vi "ATS_GetASOPC.vi"(11 "DeviceIn":i32) -> (0 "Minor":u32, 1 "Major":u32, 2 "ASoPC":string, 4 "ReturnValue":u32)   [LabVIEW 2014]
doc: "_____AlazarTech, Scope_____\n\nRetrieve the CPLG version number.\n\nInput:\n\"HandleIn\" = device to retrieve information\n\nOutput:\n\"HandleOut\" = device information\n\"Version\" = version\n\"Board\" = board name\n\"ID\" = board identification"
uses:
  ATS_ctl/ATS_Global_Ctrl.ctl
  ATS_ctl/ATS_Query.ctl
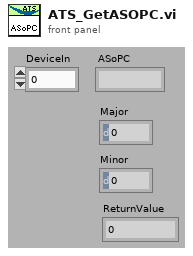
[diagram p1: front panel]
types:
  T1 = typedef "ATS_Query.ctl" = enum16{"None", "NUMBER_OF_RECORDS", "PRETRIGGER_AMOUNT", "RECORD_LENGTH", "TRIGGER_ENGINE", "TRIGGER_DELAY", "TRIGGER_TIMEOUT", "SAMPLE_RATE", "CONFIGURATION_MODE", "DATA_WIDTH", "AUTO_CALIBRATE", "TRIGGER_XXXXX", "CLOCK_SOURCE", "CLOCK_SLOPE", "IMPEDANCE", "INPUT_RANGE", "COUPLING", "MAX_TIMEOUTS_ALLOWED", "ATS_OPERATING_MODE", "CLOCK_DECIMATION_EXTERNAL", "LED_CONTROL", "ATTENUATOR_RELAY", "EXT_TRIGGER_COUPLING", "EXT_TRIGGER_ATTENUATOR_RELAY", "TRIGGER_ENGINE_SOURCE", "TRIGGER_ENGINE_SLOPE", "SEND_DAC_VALUE", "SLEEP_DEVICE", "MEMORY_SIZE", "BOARD_TYPE", "ASOPC_TYPE", "SERIAL_NUMBER", "FIRSTCAL_DATE", "LATEST_CAL_DATE", "LATEST_TEST_DATE"}
  T2 = typedef "ATS_Global_Ctrl.ctl" = enum16{"Init_Device", "Clear_ALL", "Set", "Get"}
  T3 = typedef "Device_Info.ctl" = cluster{"Handle":u32, "Board":string, "CPLD":string, "MemorySize":u32, "SampleSize":u8, "ID":i32, "High_Memory":bool, "Chan/Board":u8}
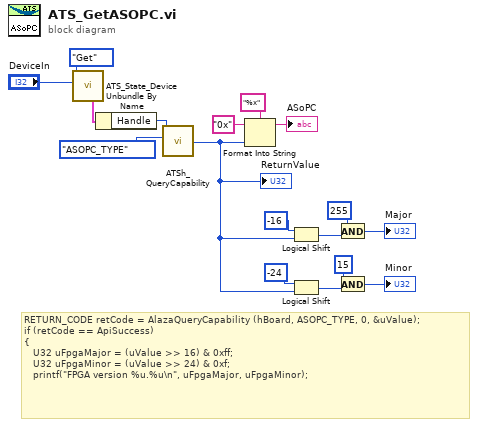
[diagram p0: block diagram]
diagram:
  # "RETURN_CODE retCode = AlazaQueryCapability (hBoard, ASOPC_TYPE, 0, &uValue);\nif (retCode == ApiSuccess)\n{\n   U32 uFpgaMajor = (uValue >> 16) & 0xff;\n   U32 uFpgaMinor = (uValue >> 24) & 0xf;\n   printf(\"FPGA version %u.%u\\n\", uFpgaMajor, uFpgaMinor);"
  n1 = call "ATS_State_Device.vi"("DeviceIn"="DeviceIn", "ATS_GBL_Ctrl"=ATS_Global_Ctrl."Get") -> ("DevInfo_Out"=w16:T3)  [unwired: 4 in, 5 out]
  n2 = Unbundle By Name(w16) -> ("Handle"=w15:u32)
  n3 = call "ATSh_QueryCapability.vi"("ATS_Query"=ATS_Query."ASOPC_TYPE", "HandleIn"=w15) -> ("ReturnValue"=w2:u32)  [unwired: 6 in, 3 out]
  "ReturnValue" <- w2
  n4 = Format Into String(format string="%x", initial string="0x", w2) -> (resulting string=→"ASoPC":string)  [unwired: 1 in, 1 out]
  n5 = Logical Shift(y=i16 -16, x=w2) -> (x << y=w4:u32)
  n6 = Logical Shift(y=i16 -24, x=w2) -> (x << y=w8:u32)
  n7 = And(x=u32 255, y=w4) -> (x .and. y?=→"Major":u32)
  n8 = And(x=u32 15, y=w8) -> (x .and. y?=→"Minor":u32)
